vi "Initialize (bundle settings and connect).vi"(8 "error in (no error)":errorcluster, 10 "Stage Comms":T1={"CommsProtocol.lvclass"=refnum, "CommsProtocol.lvclass 2"=refnum, "CommsProtocol.lvclass 3"=refnum, "XYZ Control Config"=enum."XYZ", "Translation Stage Description"=""}, 11 "Scientifica XYZ Gen1 in":refnum<class "Scientifica XYZ Gen1.lvclass">) -> (0 "error out":errorcluster, 3 "Scientifica XYZ Gen1 out":refnum<class "Scientifica XYZ Gen1.lvclass">)   [LabVIEW 2020, in "TranslationStageClassStructure.lvlib" / "Scientifica XYZ Gen1.lvclass"]
uses:
  Scientifica XYZ Gen1.lvclass
  typedefs/TranslationStageControlInfo.ctl
  Generic Comms/CommsProtocol/CommsProtocol.lvclass
  typedefs/XYZControlConfig.ctl
  Serial Comms/Serial - Settings.ctl
  Serial Comms/Serial Comms/Serial Comms.lvclass
  Serial Comms/Serial Comms/Serial Comms.lvclass/Serial Comms.ctl
  Scientifica XYZ Gen1.lvclass/Scientifica XYZ Gen1.ctl
  Serial Comms/Serial Comms/Data Member Access/Read VISA resource name .vi
  Serial Comms/Serial Comms/Data Member Access/Read baud rate.vi
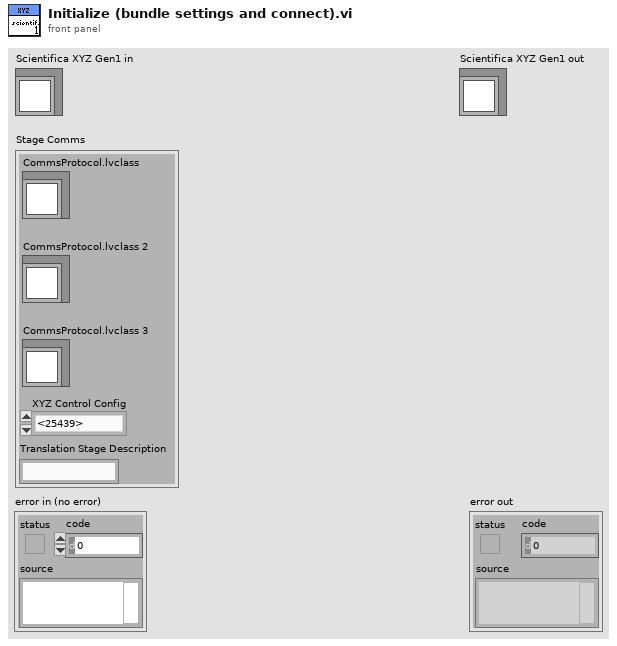
[diagram p1: front panel]
types:
  T1 = typedef "TranslationStageControlInfo.ctl" = cluster{"CommsProtocol.lvclass":refnum<class "CommsProtocol.lvclass">, "CommsProtocol.lvclass 2":refnum<class "CommsProtocol.lvclass">, "CommsProtocol.lvclass 3":refnum<class "CommsProtocol.lvclass">, "XYZ Control Config":T2, "Translation Stage Description":string}
  T2 = typedef "XYZControlConfig.ctl" = enum16{"None", "XYZ", "XY-Z", "X-Y-Z", "Z"}
  T3 = typedef "Serial - Settings.ctl" = cluster{"VISA resource name ":refnum<visa-resource-name>, "baud rate":u32, "data bits":u16, "parity":enum16{"None", "Odd", "Even", "Mark", "Space"}, "stop bits":u16, "flow control":u16, "Timeout":u32, "termination char\n(0xA = '\\n' = LF) ":u8, "Enable Termination Character":bool}
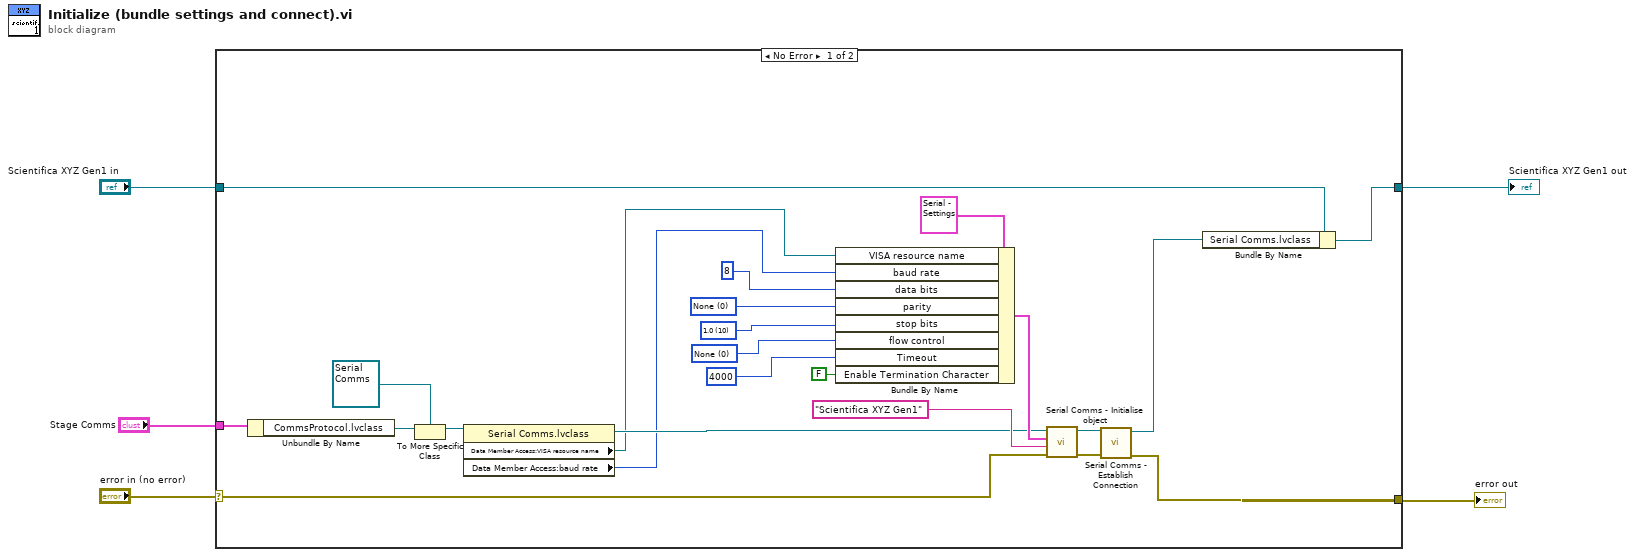
[diagram p0: block diagram]
diagram:
  n1 = case shown="No Error" "error in (no error)" {
    selector: "error in (no error)" -> [w9 w30]
    tunnel: [w8 w30] -> w4
    tunnel: [w6 w29] -> w2
    tunnel: "Scientifica XYZ Gen1 in" -> [w7 w29]
    tunnel: "Stage Comms" -> [w10 _]
    frame No Error {
      w20 = u16 0 items=["None"=0, "XON/XOFF"=1, "RTS/CTS"=2, "DTR/DSR"=4] ("flow control")
      w21 = u16 10 items=["1.0"=10, "1.5"=15, "2.0"=20] ("stop bits")
      w22 = u16 0 items=["None", "Odd", "Even", "Mark", "Space"] ("parity")
      n2 = Unbundle By Name(w10) -> ("CommsProtocol.lvclass"=w16:refnum<class "CommsProtocol.lvclass">)
      n3 = To More Specific Class(target class=refnum<class "Serial Comms.lvclass"> refnum ("Serial Comms.lvclass"), reference=w16) -> (specific class reference=w14:refnum<class "Serial Comms.lvclass">)  [unwired: 1 in, 1 out]
      n4 = property class="Serial Comms.lvclass"(reference=w14) -> (reference out=w13:refnum<class "Serial Comms.lvclass">, "Data Member Access:VISA resource name "=w12:refnum<visa-resource-name>, "Data Member Access:baud rate"=w11:u32)  [unwired: 1 in, 1 out]
      n5 = Bundle By Name(cluster=T3 {"VISA resource name "="", "baud rate"=9600, "data bits"=8, "parity"=enum."None", "stop bits"=10, "flow control"=0, "Timeout"=0, "termination char\n(0xA = '\\n' = LF) "=10, "Enable Termination Character"=FALSE} ("Serial Settings"), "VISA resource name"=w12, "baud rate"=w11, "data bits"=u16 8, "parity"=w22, "stop bits"=w21, "flow control"=w20, "Timeout"=u32 4000, "Enable Termination Character"=FALSE) -> (w24:T3)
      n6 = call "Serial Comms - Initialise object.vi"("error in (no error)"=w9, "Connection Name"="Scientifica XYZ Gen1", "Serial Settings"=w24, "Serial Comms in"=w13) -> ("error out"=w19:errorcluster, "Serial Comms out"=w18:refnum<class "Serial Comms.lvclass">)  [unwired: 6 in]
      n7 = call "Serial Comms - Establish Connection.vi"("error in (no error)"=w19, "Serial Comms in"=w18) -> ("error out"=w8:errorcluster, "Serial Comms out"=w17:refnum<class "Serial Comms.lvclass">)  [unwired: 8 in]
      n8 = Bundle By Name(cluster=w7, "Serial Comms.lvclass"=w17) -> (w6:refnum<class "Scientifica XYZ Gen1.lvclass">)
    }
    frame Error {
    }
  }
  "error out" <- w4
  "Scientifica XYZ Gen1 out" <- w2
